vi "gauss.vi"(9 "w":dbl, 10 "N2":i32, 11 "N1":i32) -> (1 "Array":dbl[][](array[numeric]), 2 "N2 2":i32, 3 "N1 out":i32)   [LabVIEW 2014]
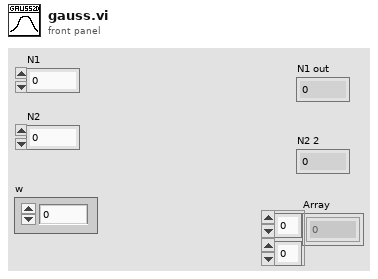
[diagram p1: front panel]
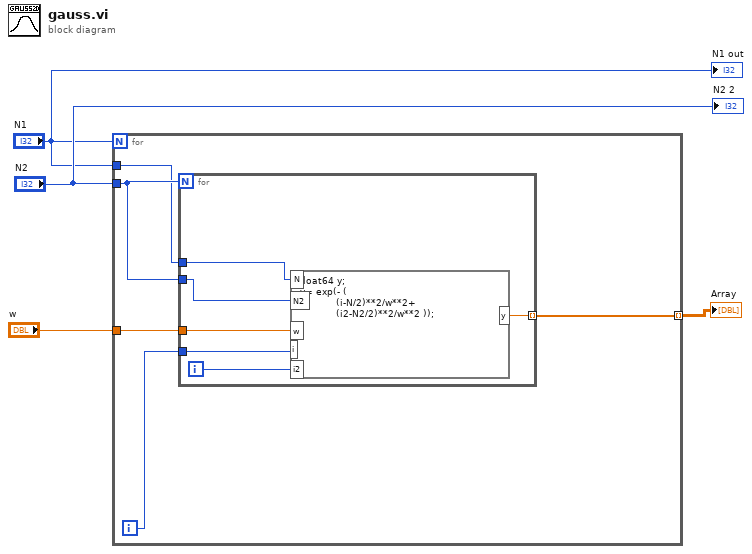
[diagram p0: block diagram]
diagram:
  n1 = for {
    N: "N1" -> [_]
    tunnel: "N1" -> [w8]
    tunnel: "N2" -> [w9]
    tunnel: "w" -> [w7]
    tunnel: [w5] -> w1 mode=indexing
    i -> [w6]
    n2 = for {
      N: w9 -> [_]
      tunnel: w9 -> [w13]
      tunnel: [w14] -> w5 mode=indexing
      tunnel: w8 -> [w12]
      tunnel: w7 -> [w11]
      tunnel: w6 -> [w10]
      i -> [w15]
      n3 = formula code="float64 y;\ny= exp(- ( \n            (i-N/2)**2/w**2+\n            (i2-N2/2)**2/w**2 ));" ("Formelknoten")("N"=w12, "w"=w11, "i2"=w15, "N2"=w13, "i"=w10) -> ("y"=w14:dbl)
    }
  }
  "Array" <- w1
  "N1 out" <- "N1"
  "N2 2" <- "N2"
